vi "mbed-read.vi"(4 "timeout (10sec)":u32=10000, 6 "Baud Rate":u32=9600, 7 "Serial Port":refnum<visa-resource-name>) -> (0 "Array of Numbers":dbl[](array[numeric]), 1 "Array of Strings":string[](array[string]), 2 "Number":dbl, 3 "Line String":string)   [LabVIEW 2009]
uses:
  <vilib>/Instr/_visa.llb/VISA Configure Serial Port (Instr).vi
panel:
  out "Status":errorcluster
  out "VISA resource name out":refnum<visa-resource-name>
  # "mbed Read"
  # "http://mbed.org"
  # "Serial Settings"
  # "Output Data"
  # "Debug"
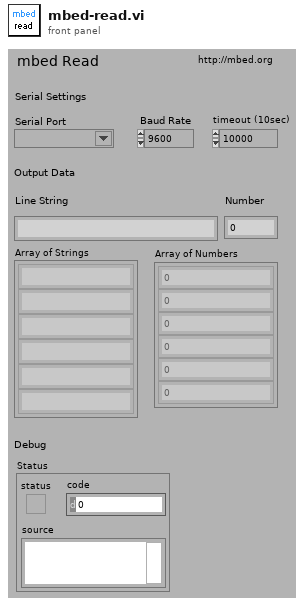
[diagram p1: front panel]
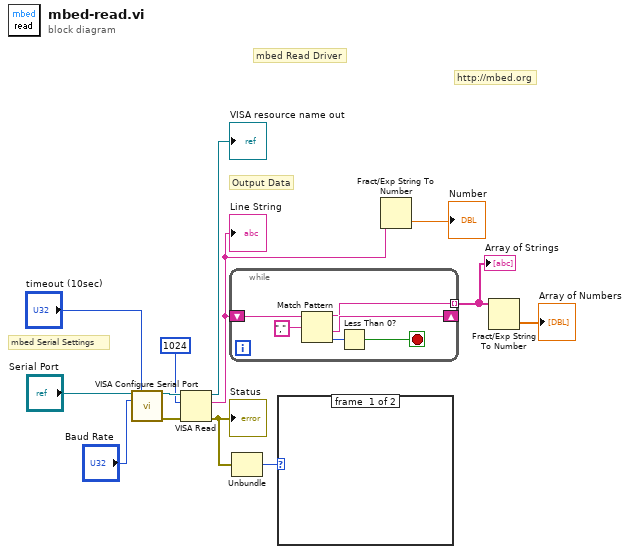
[diagram p0: block diagram]
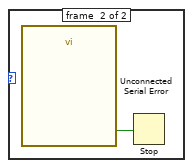
[diagram p2: hidden frame]
diagram:
  # "http://mbed.org"
  # "mbed Read Driver"
  # "Output Data"
  # "mbed Serial Settings"
  n1 = call-poly "VISA Configure Serial Port"("VISA resource name"="Serial Port", "timeout (10sec)"="timeout (10sec)", "baud rate (9600)"="Baud Rate") -> ("VISA resource name out"=w11:refnum<visa-resource-name>, "error out"=w10:errorcluster)  [unwired: 11 in]
  n2 = VISA Read(VISA resource name=w11, byte count=u32 1024, error in (no error)=w10) -> (VISA resource name out=→"VISA resource name out":refnum<visa-resource-name>, read buffer=w2:string, error out=w5:errorcluster)  [unwired: 1 out]
  "Line String" <- w2
  "Status" <- w5
  n3 = while {
    tunnel: [w16] -> w7 mode=indexing
    shift-right: [w17] -> _
    shift-left: w2 -> [w19]
    stop <- w14 stop-if-true
    n4 = Match Pattern(string=w19, regular expression=",") -> (before substring=w16:string, after substring=w17:string, offset past match=w15:i32)  [unwired: 2 out]
    n5 = Less Than 0?(x=w15) -> (x < 0?=w14:bool)
  }
  "Array of Strings" <- w7
  n6 = Unbundle(w5) -> ("code"=w4:i32)  [unwired: 2 out]
  n7 = case shown="1" w4 {
    frame #0 {
    }
    frame #1 {
      n8 = call "Unconnected Serial Error"() -> ("OK"=w20:bool)  [unwired: 10 in, 1 out]
      n9 = Stop(stop? (T)=w20) -> ()
    }
  }
  n10 = Fract/Exp String To Number(string=w2) -> (number=→"Number":dbl)  [unwired: 3 in, 1 out]
  n11 = Fract/Exp String To Number(string=w7) -> (number=→"Array of Numbers":dbl[])  [unwired: 3 in, 1 out]
